vi "Configure Output Range.vi"(6 "range (0.0)":dbl format="%^.2e", 8 "error in (no error)":errorcluster, 9 "range type (Voltage)":i32(ring)=1 items=["Voltage"=1, "Current"=0], 10 "channel name (\"CHANNEL1\")":string="CHANNEL1", 11 "CS++DCPwr in":refnum<class "CS++DCPwr.lvclass">) -> (0 "error out":errorcluster, 3 "CS++DCPwr out":refnum<class "CS++DCPwr.lvclass">)   [LabVIEW 2013, in "CS++DCPwr.lvlib" / "CS++DCPwr.lvclass"]
doc: "Configures the power supply's output range on a channel. You specify whether you want to configure the voltage or current range, and the value to which to set the range.\n\nNotes:\n\n1) Setting a voltage range can invalidate a previously configured current range.\n\n2) Setting a current range can invalidate a previously configured voltage range."
uses:
  CS++DCPwr.lvclass
  Core/Classes/CS++ProcessVariables/ProcessVariable/PV.lvclass
  Core/Classes/CS++ProcessVariables/ProcessVariable/PV.lvclass/PV.ctl
  CS++DCPwr.lvclass/CS++DCPwr.ctl
  Core/Classes/CS++ProcessVariables/PVConnection/PVConnection.lvclass
  Core/Classes/CS++ProcessVariables/ProcessVariable/Write Data.vi
  Core/Classes/CS++ProcessVariables/ProcessVariable/Write Timestamp.vi
  Core/Classes/CS++ProcessVariables/ProcessVariable/Write Quality.vi
  Core/Classes/CS++ProcessVariables/ProcessVariable/Write status.vi
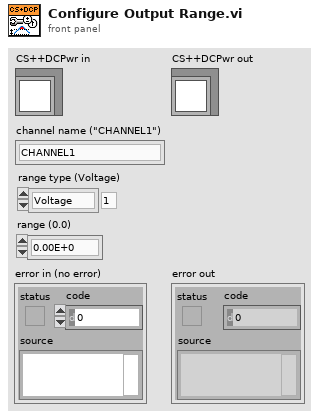
[diagram p1: front panel]
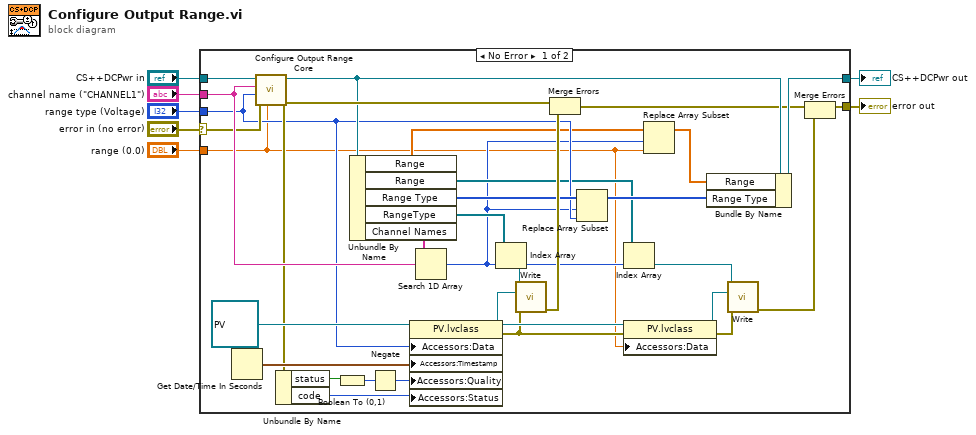
[diagram p0: block diagram]
diagram:
  n1 = case shown="No Error" "error in (no error)" {
    selector: "error in (no error)" -> [w22 w40]
    tunnel: "CS++DCPwr in" -> [w39 w41]
    tunnel: "range type (Voltage)" -> [w21 _]
    tunnel: "channel name (\"CHANNEL1\")" -> [w28 _]
    tunnel: [w10 w40] -> w5
    tunnel: [w25 w41] -> w6
    tunnel: "range (0.0)" -> [w14 _]
    frame No Error {
      n2 = Get Date/Time In Seconds() -> (seconds since 1Jan1904=w38:timestamp)
      n3 = call-dynamic "Configure Output Range Core.vi"("range (0.0)"=w14, "error in (no error)"=w22, "range type (Voltage)"=w21, "channel name (\"CHANNEL1\")"=w28, "CS++DCPwr in"=w39) -> ("error out"=w27:errorcluster, "CS++DCPwr out"=w26:refnum<class "CS++DCPwr.lvclass">)  [unwired: 5 in]
      n4 = Unbundle By Name(w27) -> ("status"=w32:bool, "code"=w30:i32)
      n5 = Boolean To (0,1)(Boolean=w32) -> (0, 1=w31:i16)
      n6 = Unbundle By Name(w26) -> ("Range"=w20:dbl[], "Range"=w18:refnum<class "PVConnection.lvclass">[], "Range Type"=w24:i32[], "RangeType"=w35:refnum<class "PVConnection.lvclass">[], "Channel Names"=w36:string[])
      n7 = Negate(x=w31) -> (-x=w29:i16)
      n8 = property class="PV.lvclass"(reference=refnum<class "PV.lvclass"> refnum ("PV"), "Accessors:Data"=w21, "Accessors:Timestamp"=w38, "Accessors:Quality"=w29, "Accessors:Status"=w30) -> (reference out=w16:refnum<class "PV.lvclass">, error out=w15:errorcluster)  [unwired: 1 in]
      n9 = Search 1D Array(1D array=w36, element=w28) -> (index of element=w17:i32)  [unwired: 1 in]
      n10 = Index Array(array=w35, index=w17) -> (element=w34:refnum<class "PVConnection.lvclass">)
      n11 = call-dynamic "Write.vi"("error in (no error)"=w15, "PV"=w16, "PVConnection in"=w34) -> ("error out"=w33:errorcluster)  [unwired: 7 in, 1 out]
      n12 = Merge Errors(w27, w33) -> (w9:errorcluster)
      n13 = Replace Array Subset(array=w24, new element=w21, index=w17) -> (w23:i32[])
      n14 = Index Array(array=w18, index=w17) -> (element=w13:refnum<class "PVConnection.lvclass">)
      n15 = property class="PV.lvclass"(reference=w16, error in=w15, "Accessors:Data"=w14) -> (reference out=w12:refnum<class "PV.lvclass">, error out=w11:errorcluster)
      n16 = Replace Array Subset(array=w20, new element=w14, index=w17) -> (w19:dbl[])
      n17 = Bundle By Name(cluster=w26, "Range"=w19, "Range Type"=w23) -> (w25:refnum<class "CS++DCPwr.lvclass">)
      n18 = call-dynamic "Write.vi"("error in (no error)"=w11, "PV"=w12, "PVConnection in"=w13) -> ("error out"=w8:errorcluster)  [unwired: 7 in, 1 out]
      n19 = Merge Errors(w9, w8) -> (w10:errorcluster)
    }
    frame Error {
    }
  }
  "error out" <- w5
  "CS++DCPwr out" <- w6
